vi "ESA-C Connect.vi"(3 "Remote=F /Local=T":bool, 4 "Drive Connection Settings":T1={"Objective GPIB-Port"=4, "Stage GPIB-Port"=4, "Drive Selector"=0, "Drive Velocity (V/s)"=5.0} {"Drive Velocity (V/s)" min=10.0 max=160.0 step=0.1 format="%.1f"; "Drive Selector" items=["Obj.", "Stage"]; "Stage GPIB-Port" min=1 max=20 step=1 format="%#.0f"; "Objective GPIB-Port" min=1 max=20 step=1 format="%#.0f"}) -> (1 "Success":bool)   [LabVIEW 2010]
uses:
  TypeDefs/ESA-C Connection Settings.ctl
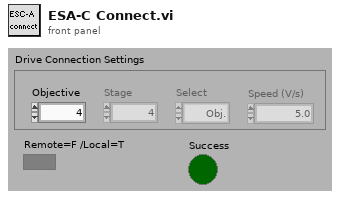
[diagram p1: front panel]
types:
  T1 = typedef "ESA-C Connection Settings.ctl" = cluster{"Objective GPIB-Port":i32, "Stage GPIB-Port":i32, "Drive Selector":u16, "Drive Velocity (V/s)":dbl}
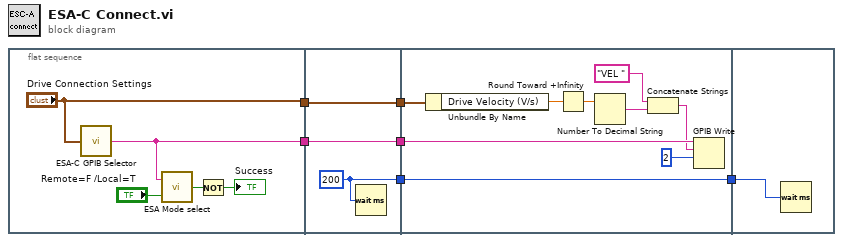
[diagram p0: block diagram]
diagram:
  n1 = flat-sequence {
    tunnel: [w8] -> w6
    tunnel: ["Drive Connection Settings"] -> w1
    tunnel: w6 -> [w14]
    tunnel: [w14] -> w5
    tunnel: [w13] -> w3
    tunnel: [w12] -> w2
    tunnel: w1 -> [w12]
    tunnel: w5 -> [w22]
    tunnel: [w17] -> w4
    tunnel: w3 -> [w17]
    tunnel: w2 -> [w16]
    tunnel: w4 -> [w24]
    frame #0 {
      n2 = call "ESA-C GPIB Selector.vi"("Drive Connection Settings"="Drive Connection Settings") -> ("String"=w8:string)
      n3 = call "ESA Mode select.vi"("Remote=F /Local=T"="Remote=F /Local=T", "GPIB Address"=w8) -> ("Status"=w10:bool)
      n4 = Not(x=w10) -> (.not. x?=→"Success":bool)
    }
    frame #1 {
      w13 = u32 200 ("Zu wartende ms")
      n5 = Wait (ms)(milliseconds to wait=w13) -> ()  [unwired: 1 out]
    }
    frame #2 {
      n6 = Unbundle By Name(w16) -> ("Drive Velocity (V/s)"=w15:dbl)
      n7 = Round Toward +Infinity(x=w15) -> (ceil(x): smallest int >= x=w21:dbl)
      n8 = Number To Decimal String(number=w21) -> (decimal integer string=w20:string)  [unwired: 1 in]
      n9 = Concatenate Strings("VEL ", w20) -> (w18:string)
      n10 = GPIB Write(0:w22, 1:w18, 2:2) -> ()  [unwired: 2 in, 2 out]
    }
    frame #3 {
      n11 = Wait (ms)(milliseconds to wait=w24) -> ()  [unwired: 1 out]
    }
  }
